vi "OFDM-SIM-A接收机.vi"(0 "input complex waveform":cluster{"t0":dbl, "dt":dbl, "Y":cdb[]}, 5 "?":T1={"过采样因子"=20.0, "脉冲成形参数"={"调制类型"=enum."PSK", "脉冲成形滤波器"=enum."Raised Cosine", "滤波器参数"=0.5, "滤波长度 (码元)"=8.0}, "载波数"=128, "总比特数"=25600, "循环次数"=100, "信噪比门限/dB"=50, "M-QAM (16)"=4} {"脉冲成形参数"."滤波器参数" format="%.2f"}, 7 "信噪比":dbl, 9 "M-QAM":i32=4 caption="M-QAM (16)", 11 "error in (no error)":errorcluster, 12 "IQ采样率":dbl format="%#_13g") -> (1 "均衡后的星座图":cdb[](graph), 2 "FFT{x}":dbl[](graph), 3 "角度":dbl[](graph), 4 "输出比特流":i8[](array[numeric]), 13 "Magnitude":dbl[](graph), 14 "Phase":dbl[](graph), 15 "error out":errorcluster)   [LabVIEW 2018]
uses:
  <vilib>/Analysis/2dsp.llb/Complex FFT.vi
  <vilib>/addons/Modulation/Analog/support/Validators/mod_Fractional Resample Validate.vi
  <vilib>/addons/Modulation/Analog/support/Validators/mod_Check Flush State.vi
  <vilib>/addons/Modulation/Analog/support/mod_FractionalResampler.vi
  <vilib>/addons/Modulation/Analog/support/mod_Integer Rate Interpolation.vi
  <vilib>/addons/Modulation/Analog/support/mod_Set Error Source.vi
  <vilib>/addons/Modulation/Analog/support/Validators/mod_Validate Complex Waveform.vi
  <vilib>/addons/Modulation/Analog/support/mod_PerformResampling.vi
  <vilib>/addons/Modulation/Analog/support/Validators/mod_WFErrorHandler.vi
  <vilib>/Utility/error.llb/Error Cluster From Error Code.vi
  <vilib>/addons/Modulation/Analog/support/mod_Resampling Factors.vi
  <vilib>/addons/Modulation/Analog/support/mod_ResamplingFilter.vi
  <vilib>/addons/Modulation/Analog/support/mod_Generate Integer Interpolation Filter.vi
  <vilib>/Analysis/NI_AALPro.lvlib
  <vilib>/addons/Modulation/niAMT.lvlib
panel:
  in  "定时频偏":i32[](array[numeric])
  out "数值":i32
  in  "?":enum32{"Magnitude", "Phase", "FFT{x}", "角度"}(tab)
  in  "?":enum32{"调制参数"}(tab)
  out "未均衡的星座图":cdb[](graph)
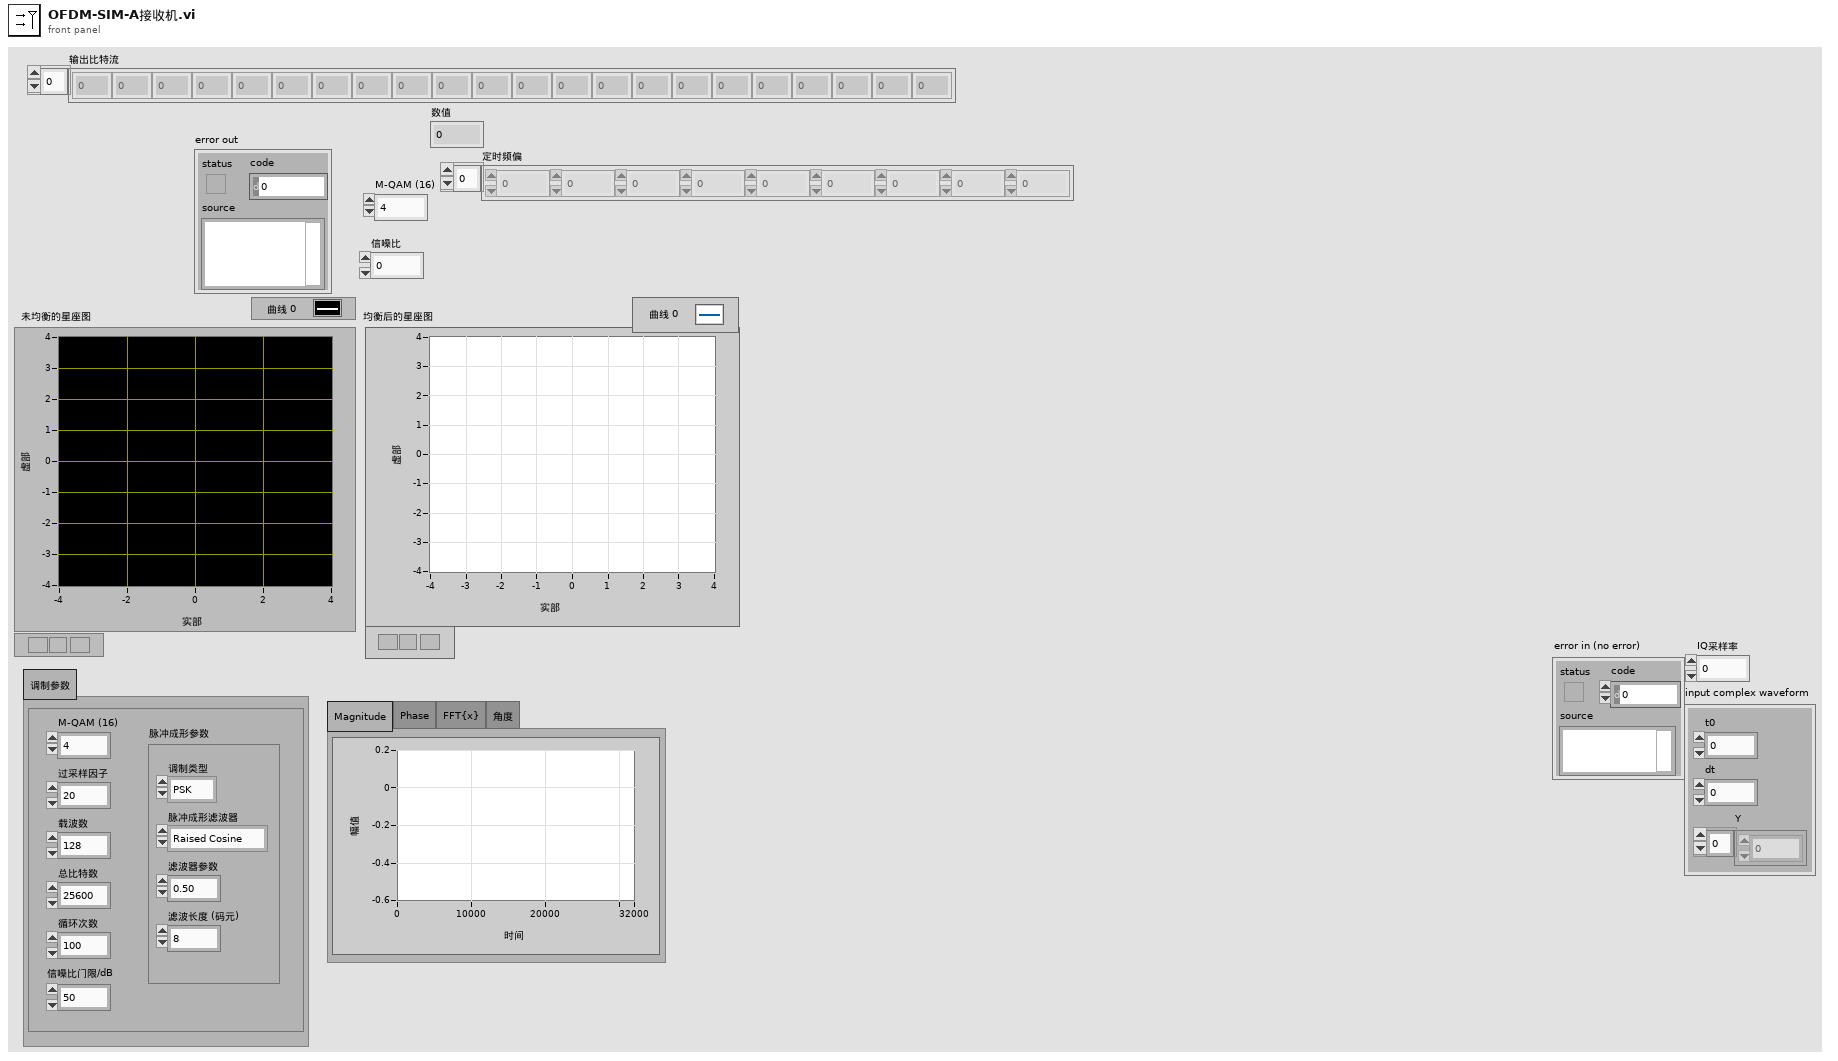
[diagram p1: front panel]
types:
  T1 = cluster{"过采样因子":dbl, "脉冲成形参数":cluster{"调制类型":enum16{"FSK", "PSK", "QAM", "MSK", "PAM", "ASK", "CPM"}, "脉冲成形滤波器":enum16{"none", "Raised Cosine", "Root Raised Cos", "Gaussian"}, "滤波器参数":dbl, "滤波长度 (码元)":dbl}, "载波数":i32, "总比特数":i32, "循环次数":i32, "信噪比门限/dB":i32, "M-QAM (16)":i32}
  T2 = typedef "niAMT.lvlib/Complex Data Waveform.ctl" = cluster{"t0":dbl, "dt":dbl, "Y":cdb[]}
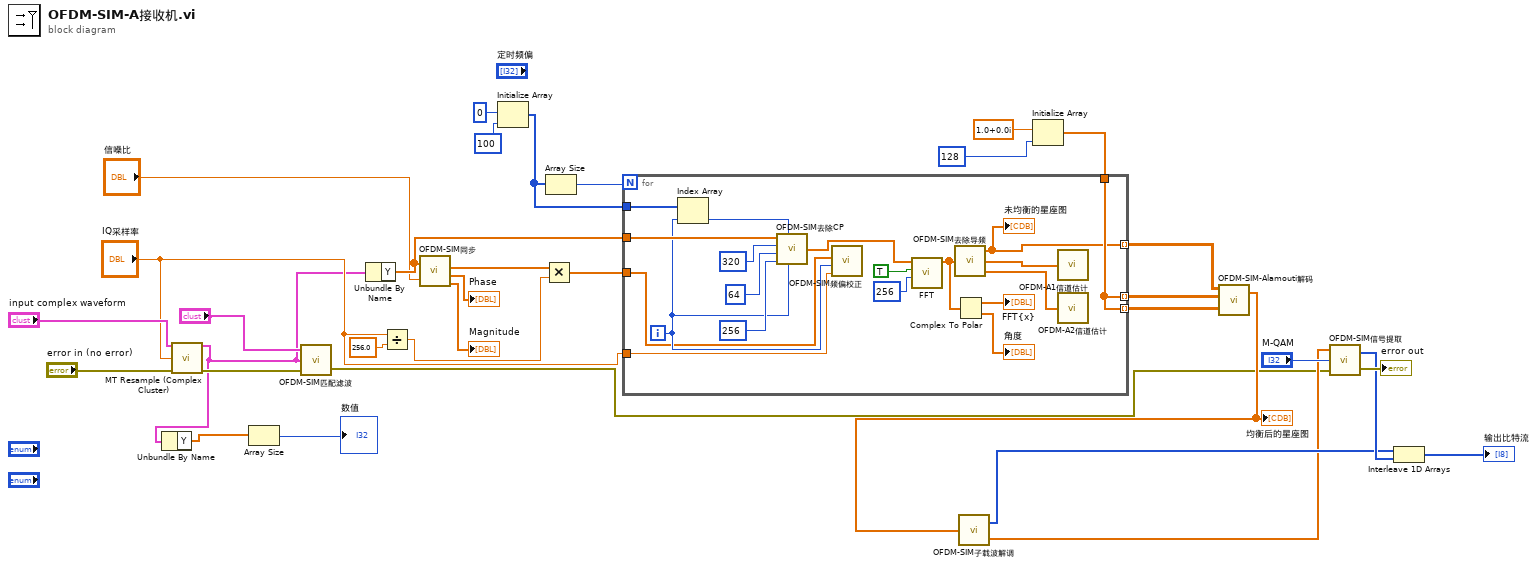
[diagram p0: block diagram]
diagram:
  n1 = call <vilib>:"MT Resample (Complex Cluster).vi"("input complex waveform"="input complex waveform", "desired sample rate (Hz)"="IQ采样率", "error in (no error)"="error in (no error)") -> ("output complex waveform"=w5:T2, "error out"=w27:errorcluster)  [unwired: 11 in]
  n2 = Unbundle By Name(w5) -> ("Y"=w17:cdb[])
  n3 = Array Size(array=w17) -> (size(s)=→"数值":i32)
  n4 = call "OFDM-SIM匹配滤波.vi"("error in (no error)"=w27, "input complex waveform"=w5, 4:"?") -> ("error out"=w6:errorcluster)  [unwired: 1 out]
  n5 = Unbundle By Name(w5) -> ("Y"=w28:cdb[])
  n6 = Divide(x="IQ采样率", y=256.0) -> (x/y=w32:dbl)
  n7 = call "OFDM-SIM同步.vi"("接收的串行数据流"=w28, "信噪比"="信噪比") -> ("频率偏移(Hz)"=w34:dbl[], "相位"=→"Phase":dbl[], "幅度"=→"Magnitude":dbl[])  [unwired: 1 out]
  n8 = Initialize Array(0, 100) -> (w15:i32[])
  n9 = Multiply(x=w34, y=w32) -> (x*y=w31:dbl[])
  n10 = Array Size(array=w15) -> (size(s)=w10:i32)
  n11 = Initialize Array(cdb 1.0+0.0i, 128) -> (w3:cdb[])
  n12 = for {
    N: w10 -> [_]
    tunnel: w28 -> [w46]
    tunnel: w15 -> [w45]
    tunnel: w31 -> [w40]
    tunnel: "IQ采样率" -> [w42]
    tunnel: [w36] -> w21 mode=indexing
    tunnel: [w36] -> w22 mode=indexing
    tunnel: w3 -> [w36]
    tunnel: [w35] -> w1 mode=indexing
    i -> [w41]
    n13 = Index Array(array=w45, index=w41) -> (element=w43:i32)
    n14 = call "OFDM-SIM去除CP.vi"("索引"=w41, "定时频偏"=w43, "FFT大小"=256, "循环前缀大小"=64, "总子载波数"=320, "接收的串行数据流"=w46) -> ("子数组"=w37:cdb[])
    n15 = call "OFDM-SIM频偏校正.vi"("采样频率"=w42, "索引"=w41, "频偏"=w40) -> ()  [unwired: 1 in, 1 out]
    n16 = call-poly <vilib>:"FFT.vi"("FFT size"=256, "shift?"=TRUE, "X"=w37) -> ("FFT {X}"=w44:cdb[])  [unwired: 7 in, 1 out]
    n17 = call "OFDM-SIM去除导频.vi"("经过FFT的OFDM符号"=w44) -> ("除去虚子载波与导频处接收的OFDM符号"=w35:cdb[], "信道1参数"=w38:cdb[], "信道2参数"=w39:cdb[])
    "未均衡的星座图" <- w35
    n18 = Complex To Polar(r * e^(i*theta)=w44) -> (r=→"FFT{x}":dbl[], theta=→"角度":dbl[])
    n19 = call "OFDM-A1信道估计.vi"("信道1导频输入"=w38) -> ()  [unwired: 1 out]
    n20 = call "OFDM-A2信道估计.vi"("信道2导频输入"=w39) -> ()  [unwired: 1 out]
  }
  n21 = call "OFDM-SIM-Alamouti解码.vi"("信道2参数"=w21, "信道1参数"=w22, "信息符号"=w1) -> ("输出符号"=w9:cdb[])  [unwired: 1 in, 1 out]
  "均衡后的星座图" <- w9
  n22 = call "OFDM-SIM子载波解调.vi"("输出符号"=w9) -> ("SIM输出"=w8:i32[], "去0后符号"=w7:cdb[])
  n23 = call "OFDM-SIM信号提取.vi"("error in"=w6, "M-QAM"="M-QAM", "待解调信号"=w7) -> ("error out"=→"error out":errorcluster, "解调信号"=w12:i32[])
  n24 = Interleave 1D Arrays(w8, w12) -> (→"输出比特流":i32[])
